vi "Destroy Publish Data Events.vi"(8 "error in (no error)":errorcluster, 11 "UserEvents in":refnum<class "User Events.lvclass">) -> (0 "error out":errorcluster, 3 "UserEvents out":refnum<class "User Events.lvclass">)   [LabVIEW 2016, in "User Events.lvclass"]
uses:
  User Events.lvclass
  User Events.lvclass/User Events.ctl
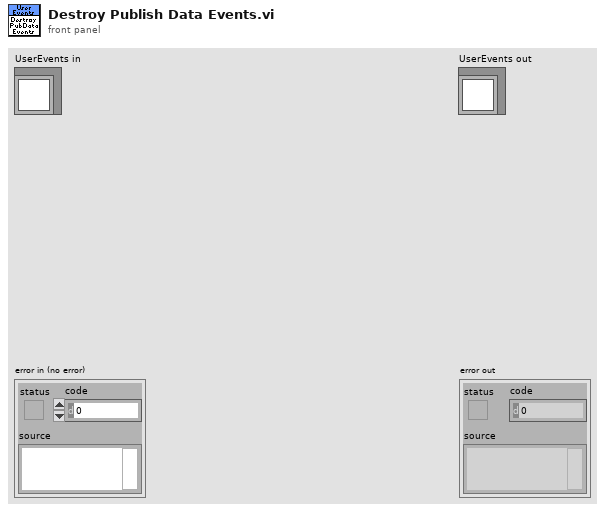
[diagram p1: front panel]
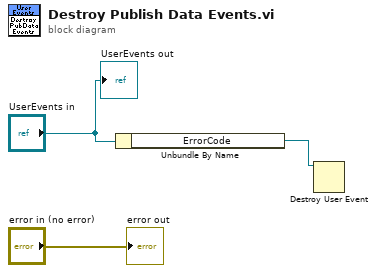
[diagram p0: block diagram]
diagram:
  n1 = Unbundle By Name("UserEvents in") -> ("ErrorCode"=w2:refnum<user-event>)
  n2 = Destroy User Event(user event=w2) -> ()  [unwired: 1 in, 1 out]
  "error out" <- "error in (no error)"
  "UserEvents out" <- "UserEvents in"
